vi "Clump to Runtime Maps.vi"(7 "Channel Data":T4[](array[typedef]), 8 "error in (no error)":errorcluster, 11 "Clumps":T1[](array[typedef])) -> (0 "error out":errorcluster, 2 "output accesses":T9[](array[typedef]), 3 "input accesses":T8[](array[typedef]))   [LabVIEW 2015]
uses:
  Output Bulk Data Access.ctl
  System Explorer/SubVIs/Modbus Type.ctl
  Shared/Controls/Data Model/Mapping.ctl
  Shared/Controls/Data Model/DataType.ctl
  <vilib>/NI Veristand/Custom Device API/Custom Device Item Ref.ctl
  Bulk Data Access.ctl
  Shared/Controls/Data Model/Channel.ctl
  <vilib>/NI Veristand/Custom Device API/Custom Device Channel Type.ctl
  clump.ctl
  Shared/Modbus Master Shared.lvlib
  <vilib>/NI VeriStand/Custom Device API/Custom Device API.lvlib
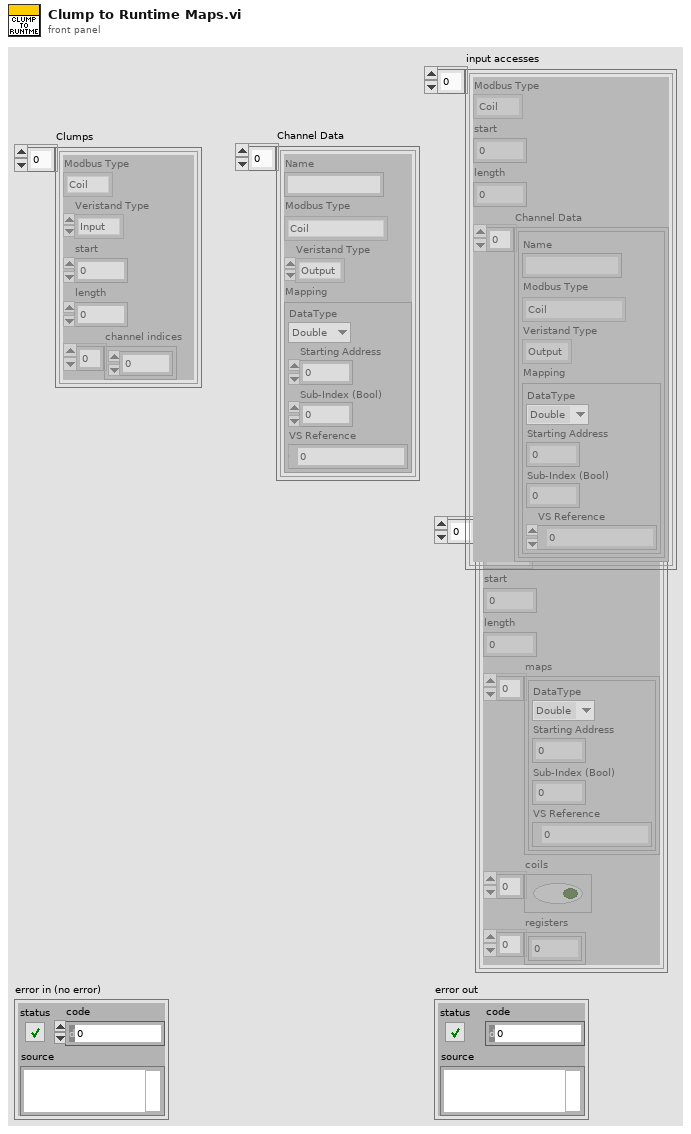
[diagram p1: front panel]
types:
  T1 = typedef "Modbus Master Shared.lvlib/clump.ctl" = cluster{"Modbus Type":T2, "Veristand Type":T3, "start":i32, "length":i32, "channel indices":i32[]}
  T2 = typedef "Modbus Master Shared.lvlib/Modbus Type.ctl" = enum16{"Coil", "Discrete Input", "Holding Register", "Input Register"}
  T3 = typedef "Custom Device API.lvlib/Custom Device Channel Type.ctl" = enum16{"Input", "Output"}
  T4 = typedef "Modbus Master Shared.lvlib/Channel.ctl" = cluster{"Name":string, "Modbus Type":T2, "Veristand Type":T3, "Mapping":T5}
  T5 = typedef "Modbus Master Shared.lvlib/Mapping.ctl" = cluster{"DataType":T6, "Starting Address":u16, "Sub-Index (Bool)":u16, "VS Reference":T7}
  T6 = typedef "Modbus Master Shared.lvlib/DataType.ctl" = enum16{"Double", "Single", "I64", "I32", "I16", "I8", "U64", "U32", "U16", "U8", "Boolean"}
  T7 = typedef "Custom Device API.lvlib/Custom Device Item Ref.ctl" = u64
  T8 = typedef "Modbus Master Shared.lvlib/Bulk Data Access.ctl" = cluster{"Modbus Type":T2, "start":u16, "length":u16, "Channel Data":T4[]}
  T9 = typedef "Modbus Master Shared.lvlib/Output Bulk Data Access.ctl" = cluster{"Modbus Type":T2, "start":u16, "length":u16, "maps":T5[], "coils":bool[], "registers":u16[]}
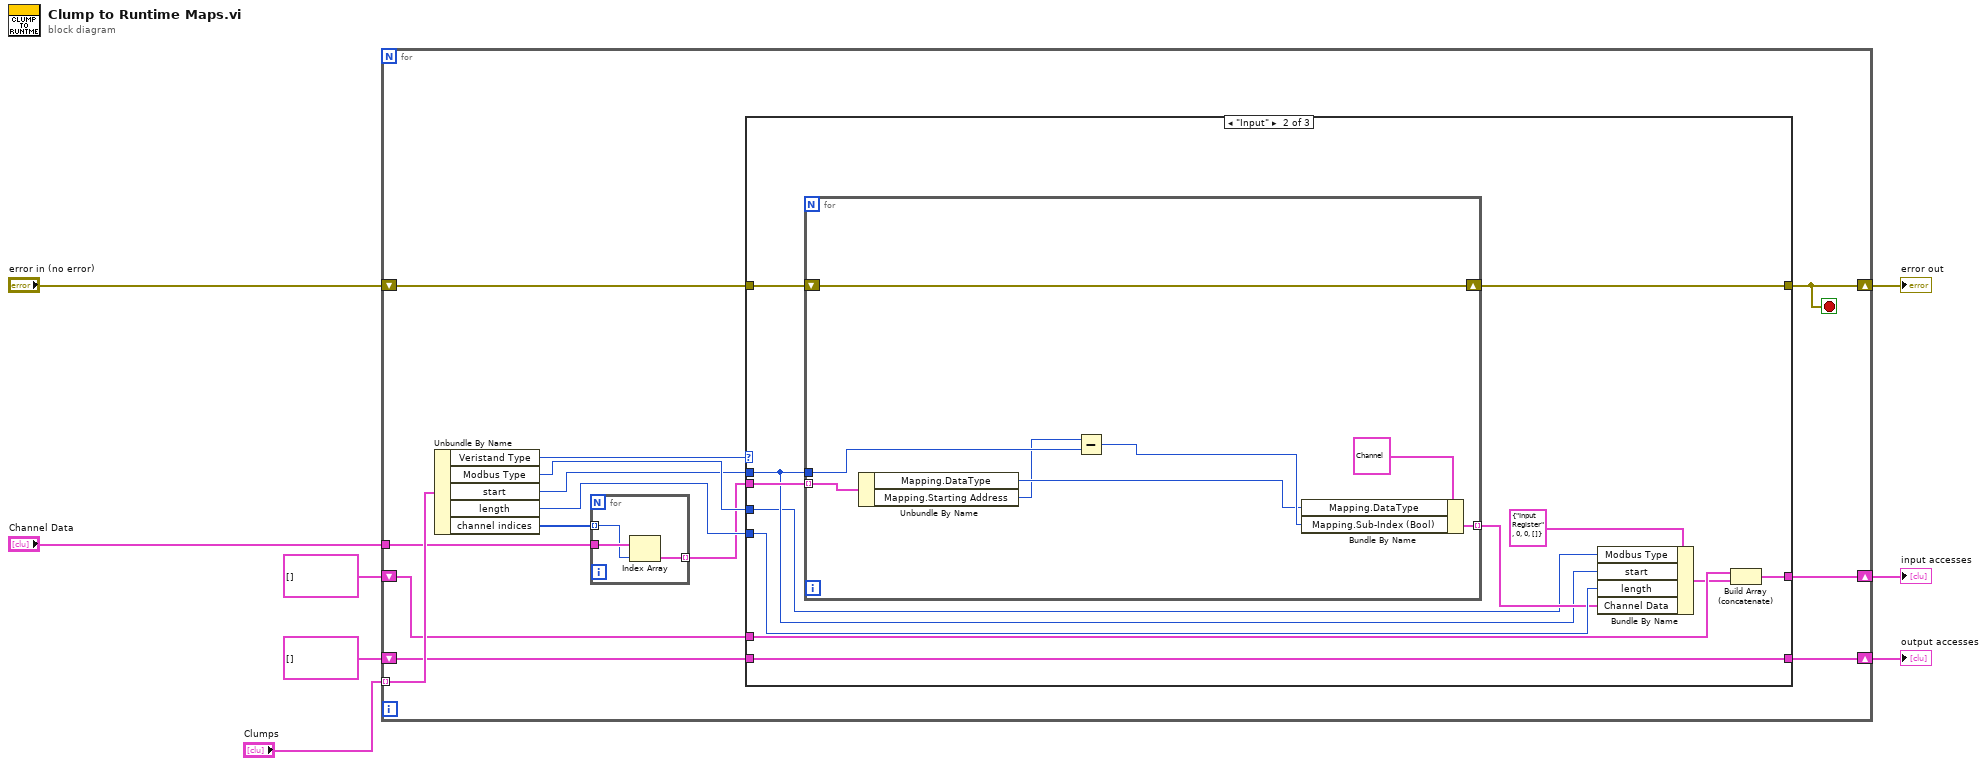
[diagram p0: block diagram]
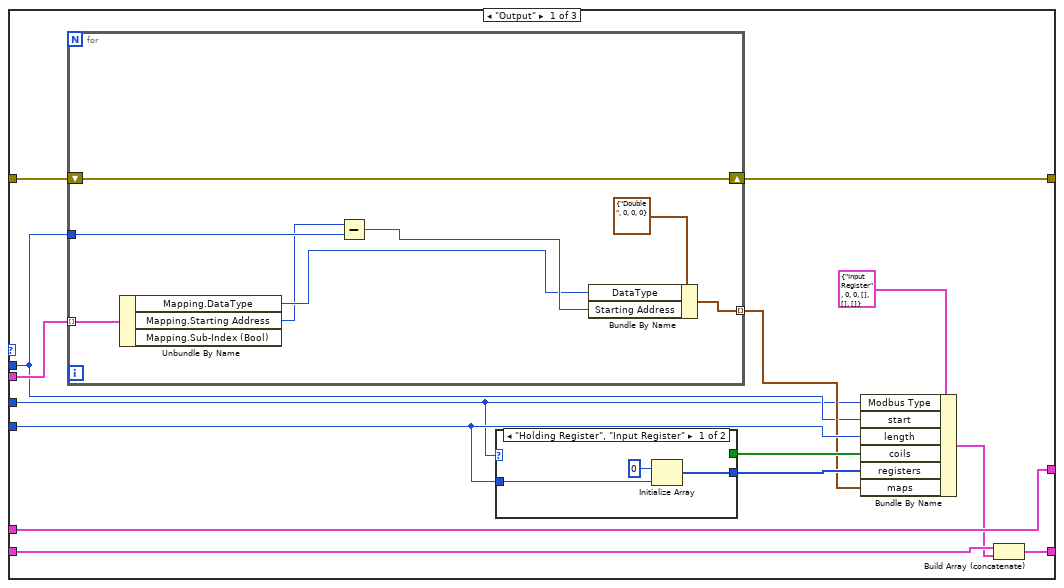
[diagram p2: hidden frame]
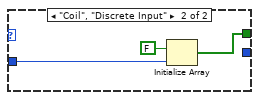
[diagram p3: hidden frame]
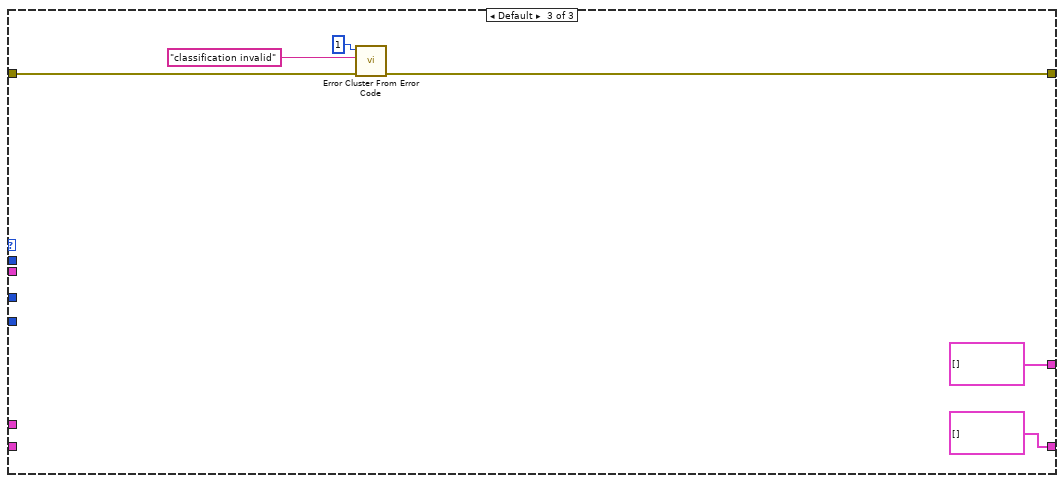
[diagram p4: hidden frame]
diagram:
  n1 = for {
    tunnel: "Clumps" -> [w22] mode=indexing
    shift-right: [w17] -> w2
    shift-left: "error in (no error)" -> [w18]
    shift-right: [w19] -> w7
    shift-left: T8[] [] ("input accesses") -> [w15]
    shift-right: [w20] -> w8
    shift-left: T9[] [] ("output accesses") -> [w16]
    tunnel: "Channel Data" -> [w9]
    stop <- w17 stop-if-true
    n2 = Unbundle By Name(w22) -> ("Veristand Type"=w21:T3, "Modbus Type"=w14:T2, "start"=w13:i32, "length"=w12:i32, "channel indices"=w11:i32[])
    n3 = for {
      tunnel: w9 -> [w79]
      tunnel: w11 -> [w78] mode=indexing
      tunnel: [w77] -> w10 mode=indexing
      n4 = Index Array(array=w79, index=w78) -> (element=w77:T4)
    }
    n5 = case shown="\"Input\"" w21 {
      tunnel: [w34 w61 T9[] [] ("output accesses")] -> w20
      tunnel: [w36 w55 T8[] [] ("input accesses")] -> w19
      tunnel: [w27 w58 w73] -> w17
      tunnel: w18 -> [w28 w59 w74]
      tunnel: w16 -> [w35 w61 _]
      tunnel: w15 -> [w36 w62 _]
      tunnel: w14 -> [w23 w53 _]
      tunnel: w13 -> [w24 w54 _]
      tunnel: w12 -> [w31 w60 _]
      tunnel: w10 -> [w25 w56 _]
      frame "Output" {
        n6 = for {
          shift-right: [w37] -> w27
          shift-left: w28 -> [w37]
          tunnel: [w41] -> w26 mode=indexing
          tunnel: w25 -> [w40] mode=indexing
          tunnel: w24 -> [w44]
          n7 = Unbundle By Name(w40) -> ("Mapping.DataType"=w39:T6, "Mapping.Starting Address"=w38:u16)  [unwired: 1 out]
          n8 = Subtract(x=w38, y=w44) -> (x-y=w42:i32)
          n9 = Bundle By Name(cluster=T5 {"DataType"=enum."Double", "Starting Address"=0, "Sub-Index (Bool)"=0, "VS Reference"=0} ("Mapping"), "DataType"=w39, "Starting Address"=w42) -> (w41:T5)
        }
        n10 = case shown="\"Holding Register\", \"Input Register\"" w23 {
          tunnel: w31 -> [w45 w50]
          tunnel: [_ w48] -> w30
          tunnel: [w47 _] -> w29
          frame "Holding Register", "Input Register" {
            n11 = Initialize Array(u16 0, w45) -> (w47:u16[])
          }
          frame "Coil", "Discrete Input" {
            n12 = Initialize Array(FALSE, w50) -> (w48:bool[])
          }
        }
        n13 = Bundle By Name(cluster=T9 {"Modbus Type"=enum."Input Register", "start"=0, "length"=0, "maps"=[], "coils"=[], "registers"=[]} ("output data access"), "Modbus Type"=w23, "start"=w24, "length"=w31, "coils"=w30, "registers"=w29, "maps"=w26) -> (w32:T9)
        n14 = Build Array (concatenate)(w35, w32) -> (w34:T9[])
      }
      frame "Input" {
        n15 = for {
          shift-right: [w64] -> w58
          shift-left: w59 -> [w64]
          tunnel: [w70] -> w57 mode=indexing
          tunnel: w56 -> [w67] mode=indexing
          tunnel: w54 -> [w68]
          n16 = Unbundle By Name(w67) -> ("Mapping.DataType"=w66:T6, "Mapping.Starting Address"=w65:u16)
          n17 = Subtract(x=w65, y=w68) -> (x-y=w69:i32)
          n18 = Bundle By Name(cluster=T4 {"Name"="", "Modbus Type"=enum."Input Register", "Veristand Type"=enum."Output", "Mapping"={"DataType"=enum."Double", "Starting Address"=0, "Sub-Index (Bool)"=0, "VS Reference"=0}} ("Channel"), "Mapping.DataType"=w66, "Mapping.Sub-Index (Bool)"=w69) -> (w70:T4)
        }
        n19 = Bundle By Name(cluster=T8 {"Modbus Type"=enum."Input Register", "start"=0, "length"=0, "Channel Data"=[]} ("output data access"), "Modbus Type"=w53, "start"=w54, "length"=w60, "Channel Data"=w57) -> (w52:T8)
        n20 = Build Array (concatenate)(w62, w52) -> (w55:T8[])
      }
      frame Default {
        n21 = call <vilib>:"Error Cluster From Error Code.vi"("error in (no error)"=w74, "error message (\"\")"="classification invalid" ("error message (\"\")"), "error code (0)"=1) -> ("error out"=w73:errorcluster)  [unwired: 6 in]
      }
    }
  }
  "output accesses" <- w8
  "input accesses" <- w7
  "error out" <- w2
